vi "multinumericlimittest2.vi"() -> (3 "Measurements":dbl[](array[numeric]))   [LabVIEW 2011]
doc: "Simulates measuring four values, then passes the results back through the VI connector pane"
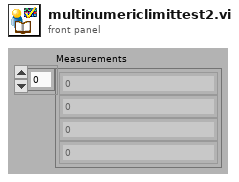
[diagram p1: front panel]
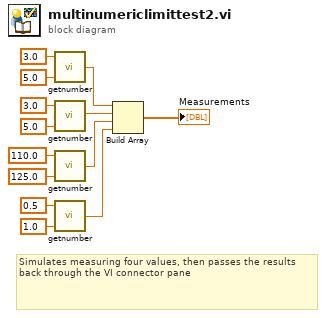
[diagram p0: block diagram]
diagram:
  # "Simulates measuring four values, then passes the results back through the VI connector pane"
  n1 = call "getnumber.vi"("High Limit"=5.0, "Low Limit"=3.0) -> ("Random Number within Limits"=w13:dbl)  [unwired: 3 out]
  n2 = call "getnumber.vi"("High Limit"=5.0, "Low Limit"=3.0) -> ("Random Number within Limits"=w10:dbl)  [unwired: 3 out]
  n3 = call "getnumber.vi"("High Limit"=125.0, "Low Limit"=110.0) -> ("Random Number within Limits"=w7:dbl)  [unwired: 3 out]
  n4 = call "getnumber.vi"("High Limit"=1.0, "Low Limit"=0.5) -> ("Random Number within Limits"=w2:dbl)  [unwired: 3 out]
  n5 = Build Array(w13, w10, w7, w2) -> (→"Measurements":dbl[])
